vi "Unbundle and Calc LG.vi"(8 "error in (no error)":errorcluster, 9 "SLM Params":T1 {"Centre X" format="%.3g"; "Centre Y" format="%.3g"}, 10 "Spot Settings":T2, 11 "holo_init":u8[](array[numeric])) -> (0 "error out":errorcluster, 3 "LG holo":u8[](array[numeric]))   [LabVIEW 2020]
uses:
  _controls/PCIe SLM params.ctl
  <userlib>/SLM ImageGen/SLM ImageGen.lvlib
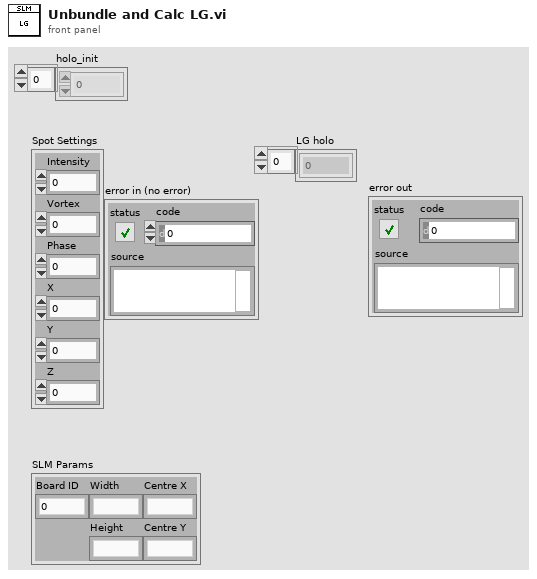
[diagram p1: front panel]
types:
  T1 = typedef "PCIe SLM params.ctl" = cluster{"Width":dbl, "Height":dbl, "Board ID":i32, "Centre Y":dbl, "Centre X":dbl}
  T2 = cluster{"Intensity":dbl, "Vortex":dbl, "Phase":dbl, "X":dbl, "Y":dbl, "Z":dbl}
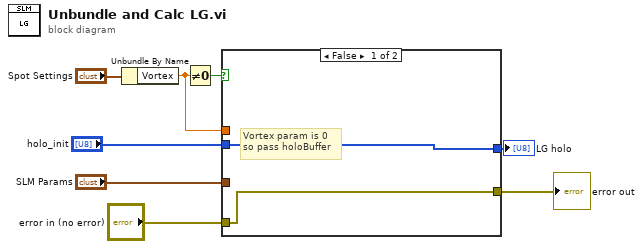
[diagram p0: block diagram]
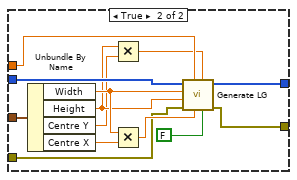
[diagram p2: hidden frame]
diagram:
  n1 = Unbundle By Name("Spot Settings") -> ("Vortex"=w7:dbl)
  n2 = Not Equal To 0?(x=w7) -> (x != 0?=w4:bool)
  n3 = case shown="False" w4 {
    tunnel: "holo_init" -> [w10 w23]
    tunnel: [w10 w22] -> w3
    tunnel: "SLM Params" -> [_ w20]
    tunnel: w7 -> [_ w19]
    tunnel: "error in (no error)" -> [w9 w12]
    tunnel: [w9 w11] -> w1
    frame False {
      # "Vortex param is 0\nso pass holoBuffer"
    }
    frame True {
      n4 = Unbundle By Name(w20) -> ("Width"=w18:dbl, "Height"=w15:dbl, "Centre Y"=w14:dbl, "Centre X"=w17:dbl)
      n5 = Multiply(x=w15, y=w14) -> (x*y=w13:dbl)
      n6 = Multiply(x=w18, y=w17) -> (x*y=w16:dbl)
      n7 = call <userlib>:"Generate LG.vi"("fork"=FALSE, "centerY"=w13, "centerX"=w16, "VortexCharge"=w19, "error in (no error)"=w12, "height"=w15, "width"=w18, "holoBuffer in"=w23) -> ("error out"=w11:errorcluster, "LG holo"=w22:u8[])  [unwired: 2 in]
    }
  }
  "LG holo" <- w3
  "error out" <- w1
